vi "LidarCommands.vi"(1 "Custom Message":u8[](array[numeric])=[2, 0, 2, 0, 32, 66, 82, 8, 2, 0, 2, 0, 32, 66, 82, 8], 2 "Message":T1(ring)) -> (0 "Output Message":u8[](array[numeric]))   [LabVIEW 2010]
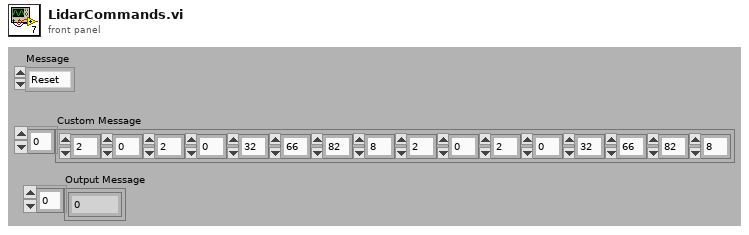
[diagram p1: front panel]
types:
  T1 = enum16{"Reset", "Set to Continous Measurement", "Change Baud to 9.6k", "Change Baud to 19.2k", "Change Baud to 38.4k", "Change Baud to 500k", "Configuration Mode", "Permanently Set Baud", "Request Status", "Custom Message"}
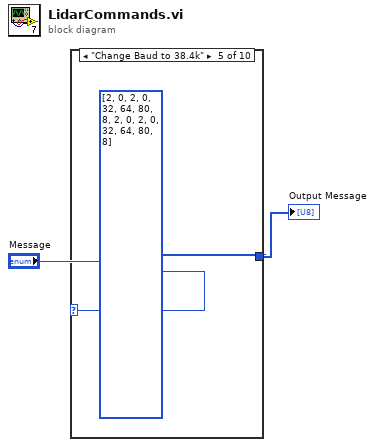
[diagram p0: block diagram]
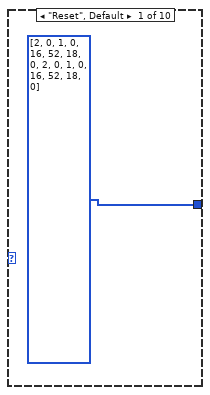
[diagram p2: hidden frame]
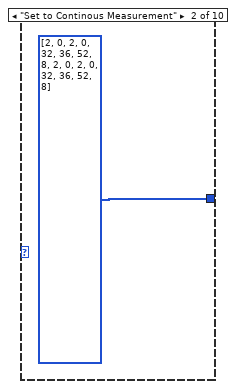
[diagram p3: hidden frame]
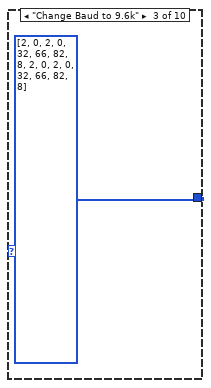
[diagram p4: hidden frame]
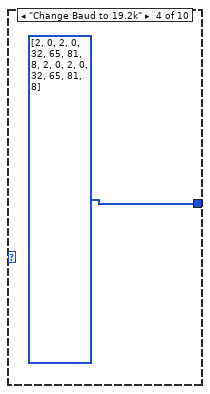
[diagram p5: hidden frame]
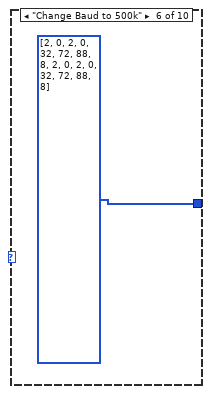
[diagram p6: hidden frame]
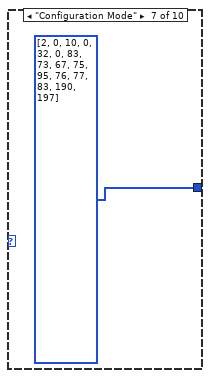
[diagram p7: hidden frame]
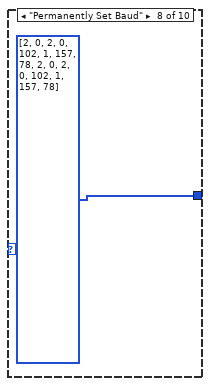
[diagram p8: hidden frame]
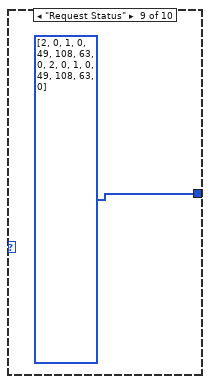
[diagram p9: hidden frame]
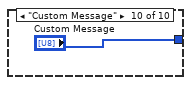
[diagram p10: hidden frame]
diagram:
  n1 = case shown="\"Change Baud to 38.4k\"" "Message" {
    tunnel: [u8[] [2, 0, 1, 0, 16, 52, 18, 0, 2, 0, 1, 0, 16, 52, 18, 0] u8[] [2, 0, 2, 0, 32, 36, 52, 8, 2, 0, 2, 0, 32, 36, 52, 8] ("start continuous measurement tellegram (repeated twice)") u8[] [2, 0, 2, 0, 32, 66, 82, 8, 2, 0, 2, 0, 32, 66, 82, 8] u8[] [2, 0, 2, 0, 32, 65, 81, 8, 2, 0, 2, 0, 32, 65, 81, 8] u8[] [2, 0, 2, 0, 32, 64, 80, 8, 2, 0, 2, 0, 32, 64, 80, 8] u8[] [2, 0, 2, 0, 32, 72, 88, 8, 2, 0, 2, 0, 32, 72, 88, 8] u8[] [2, 0, 10, 0, 32, 0, 83, 73, 67, 75, 95, 76, 77, 83, 190, 197] u8[] [2, 0, 2, 0, 102, 1, 157, 78, 2, 0, 2, 0, 102, 1, 157, 78] u8[] [2, 0, 1, 0, 49, 108, 63, 0, 2, 0, 1, 0, 49, 108, 63, 0] "Custom Message"] -> w2
    frame "Reset", Default {
    }
    frame "Set to Continous Measurement" {
    }
    frame "Change Baud to 9.6k" {
    }
    frame "Change Baud to 19.2k" {
    }
    frame "Change Baud to 38.4k" {
    }
    frame "Change Baud to 500k" {
    }
    frame "Configuration Mode" {
    }
    frame "Permanently Set Baud" {
    }
    frame "Request Status" {
    }
    frame "Custom Message" {
    }
  }
  "Output Message" <- w2
